vi "PID_2Chan_Direct_flowV2.vi"() -> ()   [LabVIEW 2016]
uses:
  <vilib>/Analysis/baseanly.llb/Mean (DBL).vi
  <vilib>/addons/control/pid/pid.llb/PID Advanced (DBL Array).vi
  <vilib>/addons/control/pid/pid.llb/PID Parameter Manager (DBL Array).vi
  <vilib>/addons/control/pid/pid.llb/PID Derivative Action Buffered (DBL Array).vi
  <vilib>/addons/control/pid/pid.llb/PID Get Advanced Error (DBL Array).vi
  <vilib>/addons/control/pid/pid.llb/PID Integral Action Buffered (DBL Array).vi
  <vilib>/addons/control/pid/pid.llb/PID Resize 1D Array.vi
  <vilib>/addons/control/pid/pid.llb/PID Get Advanced Error (DBL).vi
  <userlib>/Fluigent/Fluigent MFCS/FluigentMFCS_Full.llb/MFCS_EZ Detect.vi
  <userlib>/Fluigent/Fluigent MFCS/FluigentMFCS_Full.llb/MFCS_EZ Initialization.vi
  <userlib>/Fluigent/Fluigent MFCS/FluigentMFCS_Full.llb/MFCS_EZ Write Channel Pressure.vi
  <userlib>/Fluigent/Fluigent MFCS/FluigentMFCS_Full.llb/MFCS_EZ Close.vi
  <vilib>/addons/control/pid/NI_PID_pid.lvlib
  <vilib>/Analysis/NI_AALBase.lvlib
panel:
  in  "Set Ctr Pressure":dbl
  in  "reset Averging":bool
  in  "Sec2wait":dbl
  in  "set avg pressure to manual pressure":bool
  out "Pressures":T1(graph)
  out "Flow Rates":dbl[](array[numeric])
  out "Err Signal":T1(graph)
  in  "stop":bool
  out "Flow Rates":cluster{"Flow-Rate":dbl, "Flow-Rate":dbl}(graph)
  in  "Valves":enum16{"1", "2", "3", "4", "5", "6", "7", "8"}[](array[ring])=[enum."6", enum."7"]
  in  "Pressure Channels":i16[](array[numeric])
  in  "Manual Pressure Set":dbl[](array[numeric])
  in  "PID On":bool
  in  "reinitialize? (F)":bool
  in  "F0 Setpoint":dbl
  in  "F1 Setpoint":dbl
  in  "PID Gains":T2(array[cluster])=[{"Proportional Gain"=0.4, "Integral Time"=0.03, "Derivative Time"=0.0}, {"Proportional Gain"=0.4, "Integral Time"=0.03, "Derivative Time"=0.0}]
  in  "Add Ctrl?":bool=TRUE
  in  "Boards":enum16{"A", "B", "C"}[](array[ring])=[enum."A", enum."A"]
  in  "Valves":enum16{"1", "2", "3", "4", "5", "6", "7", "8"}[](array[ring])=[enum."5", enum."4"]
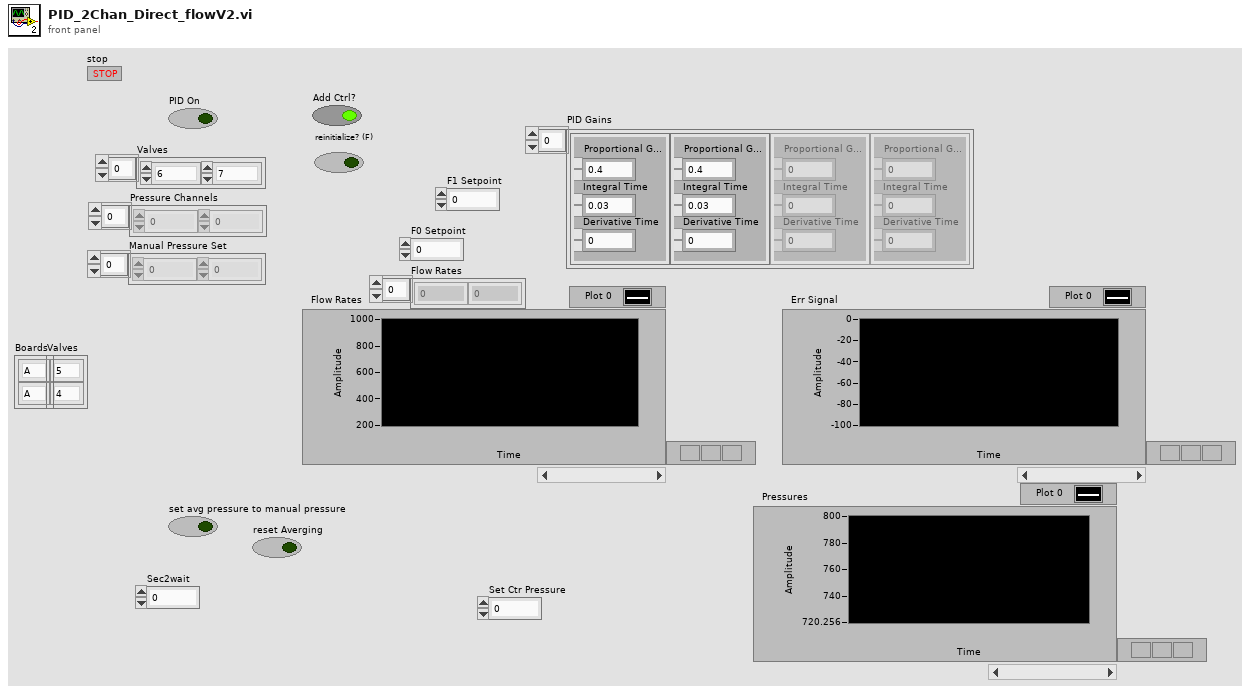
[diagram p1: front panel]
types:
  T1 = cluster{"[0]":dbl, "[1]":dbl, "[2]":dbl, "[3]":dbl, "[4]":dbl, "[5]":dbl, "[6]":dbl, "[7]":dbl, "[8]":dbl}
  T2 = cluster{"Proportional Gain":dbl, "Integral Time":dbl, "Derivative Time":dbl}[]
  T3 = typedef "_EZmfcsSN.ctl" = u16
  T4 = typedef "_EZmfcsRefNum.ctl" = refnum<k1>
  T5 = cluster{"setpoint high":dbl, "setpoint low":dbl}[]
  T6 = cluster{"output[0]":dbl, "output[1]":dbl, "output[2]":dbl, "output[3]":dbl, "output[4]":dbl, "output[5]":dbl, "output[6]":dbl, "output[7]":dbl, "output[8]":dbl}
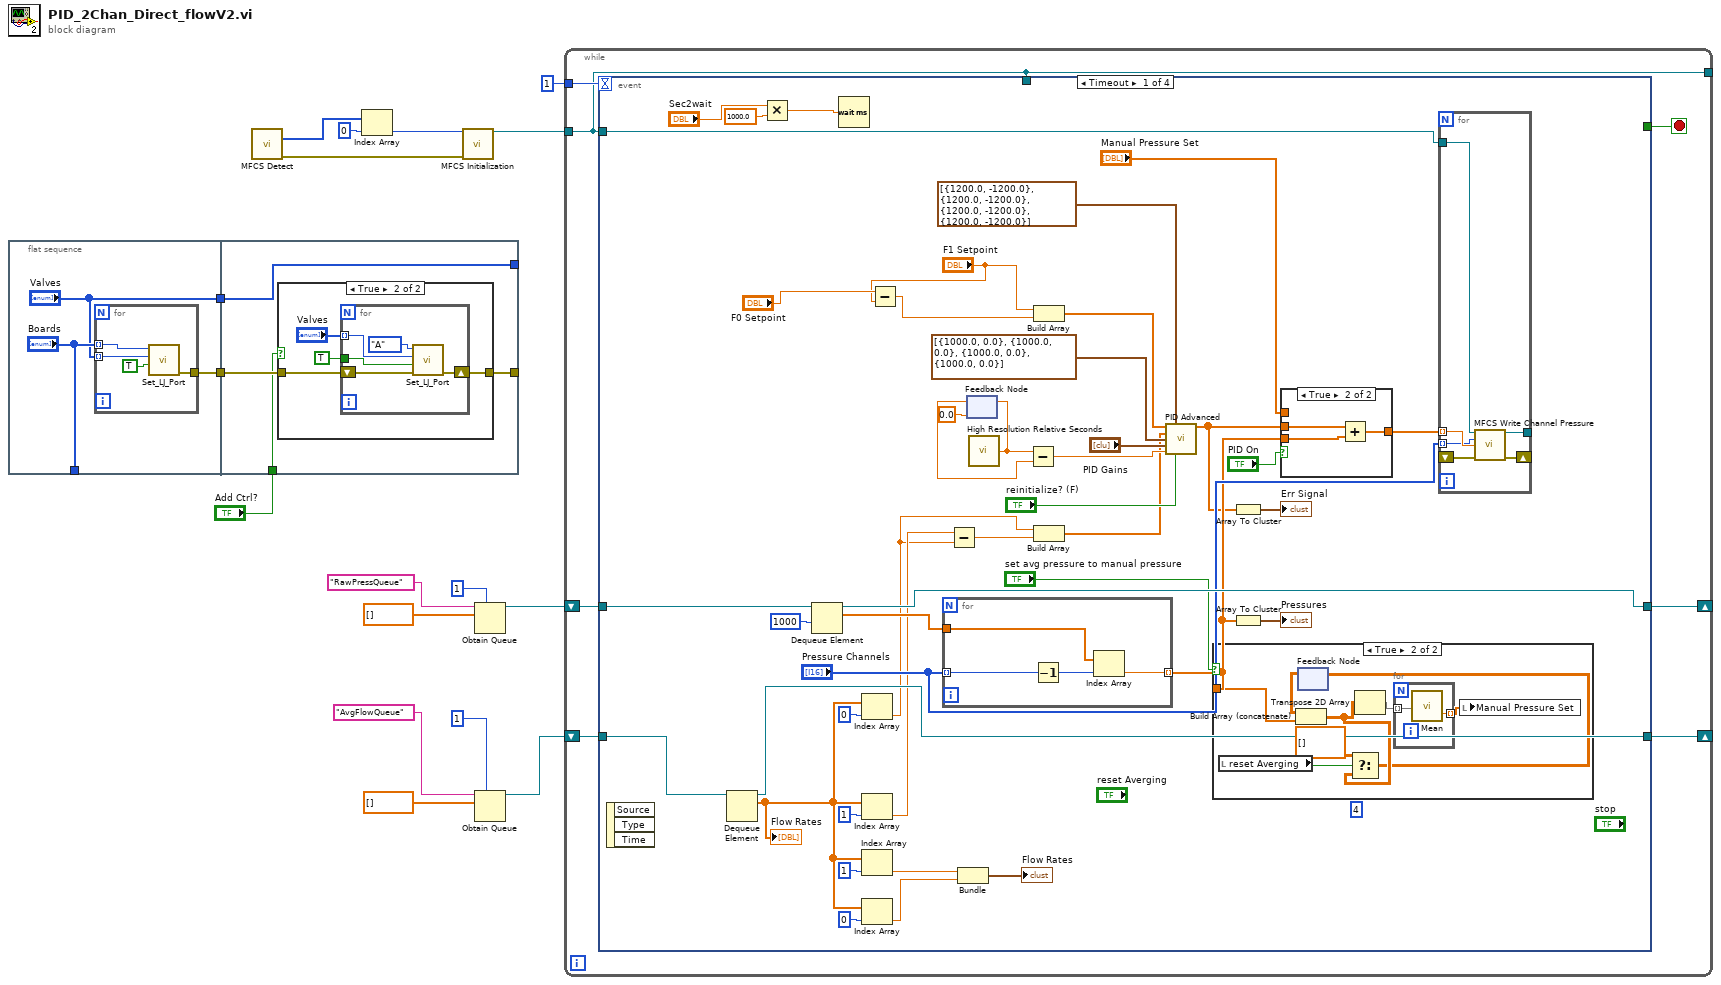
[diagram p0: block diagram]
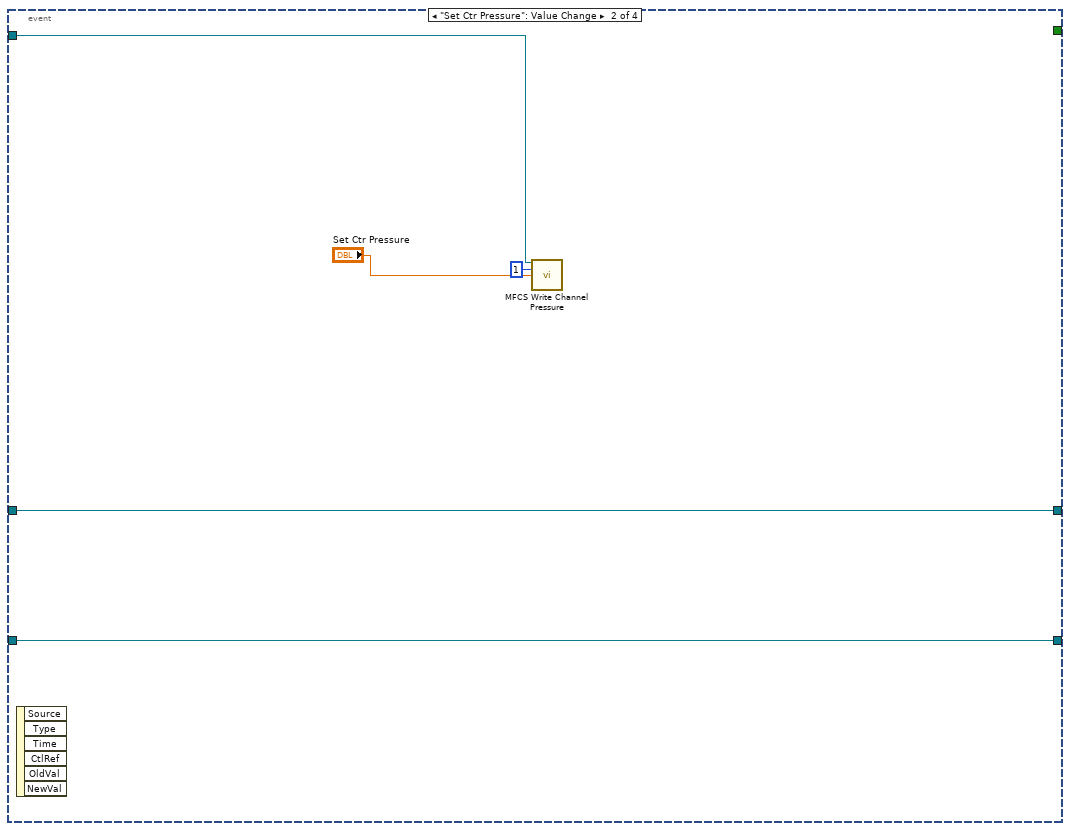
[diagram p4: hidden frame]
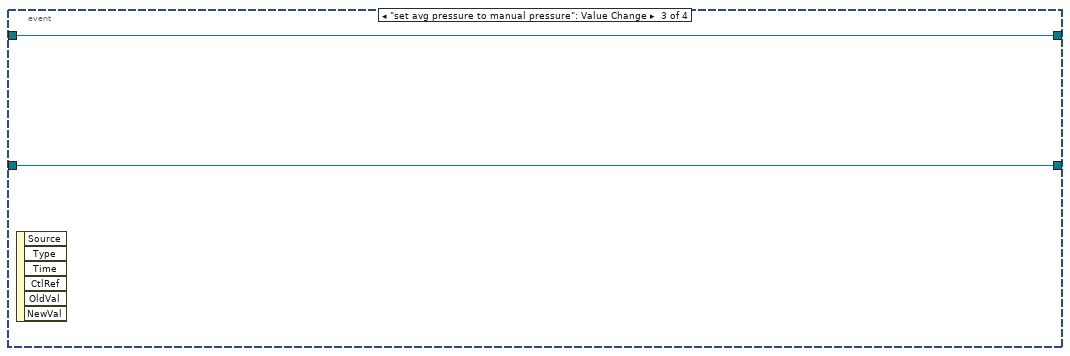
[diagram p5: hidden frame]
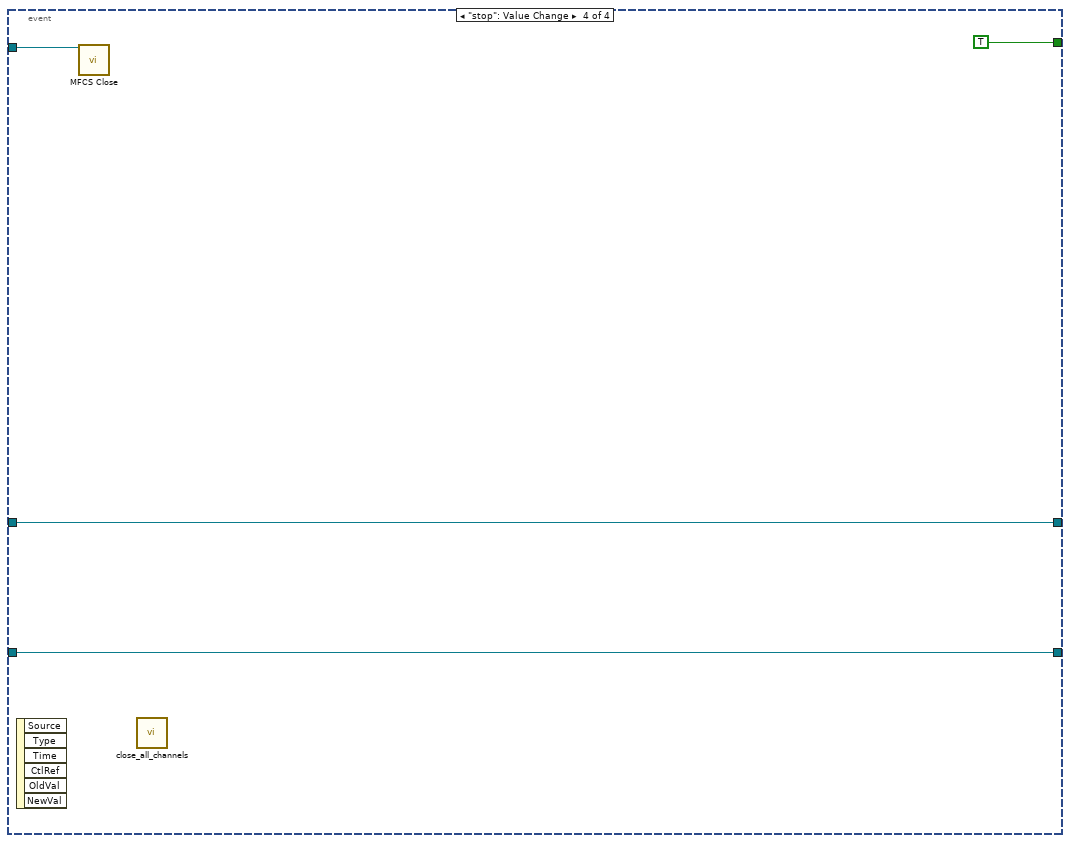
[diagram p6: hidden frame]
diagram:
  n1 = flat-sequence {
    tunnel: ["Boards"] -> _
    tunnel: [w20] -> w17
    tunnel: ["Valves"] -> w16
    tunnel: [w28] -> _
    tunnel: [w26] -> _
    tunnel: w17 -> [w27]
    tunnel: w16 -> [w28]
    tunnel: "Add Ctrl?" -> [w25]
    frame #0 {
      n2 = for {
        tunnel: "Valves" -> [w24] mode=indexing
        tunnel: "Boards" -> [w23] mode=indexing
        tunnel: [w21] -> w20
        n3 = call "Set_LJ_Port.vi"("State"=TRUE, "Channel"=w24, "Flowboard"=w23) -> ("error out"=w21:errorcluster)  [unwired: 8 in]
      }
    }
    frame #1 {
      n4 = case shown="True" w25 {
        tunnel: w27 -> [w29 w33]
        tunnel: [w29 w32] -> w26
        frame False {
        }
        frame True {
          n5 = for {
            tunnel: TRUE ("State") -> [w36]
            shift-right: [w37] -> w32
            shift-left: w33 -> [w38]
            tunnel: "Valves" -> [w35] mode=indexing
            n6 = call "Set_LJ_Port.vi"("error in"=w38, "State"=w36, "Channel"=w35, "Flowboard"=enum16{"A", "B", "C"}."A") -> ("error out"=w37:errorcluster)  [unwired: 7 in]
          }
        }
      }
    }
  }
  n7 = call-poly <userlib>:"MFCS Detect.vi"() -> ("[SN MFCS_EZ]"=w14:T3[], "error out"=w12:errorcluster)  [unwired: 14 in]
  n8 = Index Array(array=w14, index=0) -> (element=w13:T3)
  n9 = call-poly <userlib>:"MFCS Initialization.vi"("SN MFCS_EZ"=w13, "error in (no error)"=w12) -> ("MFCS_EZ"=w10:T4)  [unwired: 11 in, 2 out]
  n10 = Obtain Queue(max queue size (-1, unlimited)=1, name (unnamed)="RawPressQueue", element data type=dbl[] [] ("appended array")) -> (queue out=w2:refnum<queue>)  [unwired: 2 in, 2 out]
  n11 = Obtain Queue(max queue size (-1, unlimited)=1, name (unnamed)="AvgFlowQueue", element data type=dbl[] [] ("appended array")) -> (queue out=w3:refnum<queue>)  [unwired: 2 in, 2 out]
  n12 = while {
    tunnel: [w39] -> _
    tunnel: w10 -> [w39]
    shift-right: [w43] -> _
    shift-left: w2 -> [w44]
    shift-right: [w42] -> _
    shift-left: w3 -> [w45]
    tunnel: 1 -> [w40]
    stop <- w41 stop-if-true
    n13 = event shown="[0] Timeout" {
      selector: _ -> [_ _ _ _]
      dyn-events: _ -> [_ _ _ _]
      timeout: w40 -> [_ _ _ _]
      tunnel: w45 -> [w88 w116 w118 w120]
      tunnel: w44 -> [w87 w117 w119 w121]
      tunnel: [w86 w117 w119 w121] -> w43
      tunnel: [w85 w116 w118 w120] -> w42
      tunnel: w39 -> [w80 w115 _ w122]
      tunnel: [_ _ _ TRUE] -> w41
      tunnel: w39 -> [_ _ _ _]
      event Timeout {
        (unwired) 4 ("dimension size")
        n14 = event-data() -> ()  [unwired: 1 in, 3 out]
        n15 = Dequeue Element(queue=w88) -> (queue out=w85:refnum<queue>, element=w54:dbl[])  [unwired: 2 in, 2 out]
        "Flow Rates" <- w54
        n16 = Multiply(x="Sec2wait", y=1000.0) -> (x*y=w57:dbl)
        n17 = Dequeue Element(queue=w87, timeout in ms (-1)=1000) -> (queue out=w86:refnum<queue>, element=w63:dbl[])  [unwired: 1 in, 2 out]
        n18 = Wait (ms)(milliseconds to wait=w57) -> ()  [unwired: 1 out]
        n19 = Index Array(array=w54, index=0) -> (element=w50:dbl)
        n20 = Index Array(array=w54, index=1) -> (element=w52:dbl)
        n21 = Index Array(array=w54, index=1) -> (element=w70:dbl)
        n22 = Index Array(array=w54, index=0) -> (element=w69:dbl)
        n23 = Subtract(x="F0 Setpoint", y="F1 Setpoint") -> (x-y=w46:dbl)
        n24 = for {
          tunnel: "Pressure Channels" -> [w102] mode=indexing
          tunnel: w63 -> [w101]
          tunnel: [w99] -> w60 mode=indexing
          n25 = Decrement(x=w102) -> (x-1=w100:i16)
          n26 = Index Array(array=w101, index=w100) -> (element=w99:dbl)
        }
        n27 = Subtract(x=w52, y=w50) -> (x-y=w51:dbl)
        n28 = Bundle("Flow-Rate"=w70, "Flow-Rate"=w69) -> (→"Flow Rates":cluster{"Flow-Rate":dbl, "Flow-Rate":dbl})  [unwired: 1 in]
        n29 = feedback #1(0.0 ("relative seconds")) -> (w77:dbl)
        n30 = call <vilib>:"High Resolution Relative Seconds.vi"() -> ("relative seconds"=w76:dbl)
        n31 = feedback-in #1(w76) -> ()
        n32 = Subtract(x=w76, y=w77) -> (x-y=w75:dbl)
        n33 = Build Array("F1 Setpoint", w46) -> (w84:dbl[])
        n34 = Build Array(w50, w51) -> (w49:dbl[])
        n35 = call-poly <vilib>:"PID Advanced.vi"("setpoint"=w84, "output range"=cluster{"output high":dbl, "output low":dbl}[] [{"output high"=1200.0, "output low"=-1200.0}, {"output high"=1200.0, "output low"=-1200.0}, {"output high"=1200.0, "output low"=-1200.0}, {"output high"=1200.0, "output low"=-1200.0}], "process variable"=w49, "setpoint range"=T5 [{"setpoint high"=1000.0, "setpoint low"=0.0}, {"setpoint high"=1000.0, "setpoint low"=0.0}, {"setpoint high"=1000.0, "setpoint low"=0.0}, {"setpoint high"=1000.0, "setpoint low"=0.0}], "PID gains"="PID Gains", "dt (s)"=w75, "reinitialize? (F)"="reinitialize? (F)") -> ("output"=w56:dbl[])  [unwired: 7 in, 1 out]
        n36 = case shown="True" "set avg pressure to manual pressure" {
          tunnel: w60 -> [_ w96]
          frame False {
          }
          frame True {
            n37 = local read "reset Averging"() -> (w94:bool)
            n38 = feedback #2() -> (w95:dbl[][])  [unwired: 1 in]
            n39 = Build Array (concatenate)(w95, w96) -> (w90:dbl[][])
            n40 = Select(t=dbl[][] [] ("appended array"), s=w94, f=w90) -> (s? t:f=w89:dbl[][])
            n41 = feedback-in #2(w89) -> ()
            n42 = Transpose 2D Array(2D array=w90) -> (transposed array=w92:dbl[][])
            n43 = for {
              tunnel: w92 -> [w98] mode=indexing
              tunnel: [w97] -> w93 mode=indexing
              n44 = call-poly <vilib>:"Mean.vi"("X"=w98) -> ("mean"=w97:dbl)  [unwired: 1 out]
            }
            n45 = local write "Manual Pressure Set"(w93) -> ()
          }
        }
        n46 = Array To Cluster(array=w56) -> (cluster=→"Err Signal":T6)
        n47 = Array To Cluster(array=w60) -> (cluster=→"Pressures":T1)
        n48 = case shown="True" "PID On" {
          tunnel: "Manual Pressure Set" -> [w103 _]
          tunnel: w56 -> [_ w105]
          tunnel: w60 -> [_ w106]
          tunnel: [w103 w104] -> w73
          frame False {
          }
          frame True {
            n49 = Add(x=w105, y=w106) -> (x+y=w104:dbl[])
          }
        }
        n50 = for {
          shift-right: [w111] -> _
          shift-left: _ -> [w112]
          tunnel: [w110] -> _
          tunnel: w80 -> [w109]
          tunnel: w73 -> [w108] mode=indexing
          tunnel: "Pressure Channels" -> [w107] mode=indexing
          n51 = call-poly <userlib>:"MFCS Write Channel Pressure.vi"("MFCS_EZ"=w109, "Channel Number (default=1)"=w107, "Pressure (mBar)"=w108, "error in (no error)"=w112) -> ("MFCS_EZ out"=w110:T4, "error out"=w111:errorcluster)  [unwired: 10 in]
        }
      }
      event "Set Ctr Pressure": Value Change {
        n52 = event-data() -> ()  [unwired: 1 in, 6 out]
        n53 = call-poly <userlib>:"MFCS Write Channel Pressure.vi"("MFCS_EZ"=w115, "Channel Number (default=1)"=u8 1, "Pressure (mBar)"="Set Ctr Pressure") -> ()  [unwired: 11 in, 2 out]
      }
      event "set avg pressure to manual pressure": Value Change {
        n54 = event-data() -> ()  [unwired: 1 in, 6 out]
      }
      event "stop": Value Change {
        n55 = event-data() -> ()  [unwired: 1 in, 6 out]
        n56 = call-poly <userlib>:"MFCS Close.vi"("MFCS_EZ"=w122) -> ()  [unwired: 14 in, 1 out]
        n57 = call "close_all_channels.vi"() -> ()  [unwired: 12 in]
      }
    }
  }
